vi "test_VIRefnumArray.vi"(8 "error in (no error)":errorcluster) -> (0 "error out":errorcluster)   [LabVIEW 2020]
uses:
  run-tests/Run Test (VIRefnum Array).vi
  Caraya.lvlib
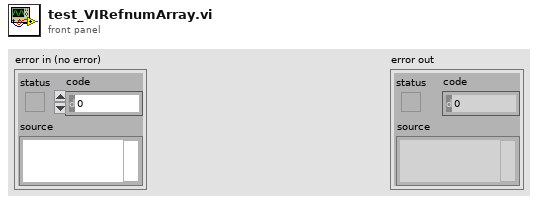
[diagram p1: front panel]
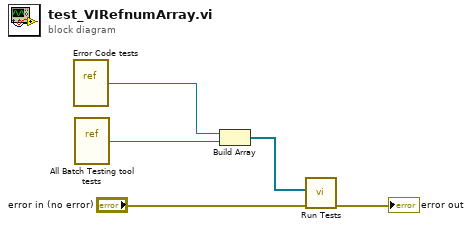
[diagram p0: block diagram]
diagram:
  n1 = vi-ref "Error Code tests.vi"() -> (w2:refnum<vi>)
  n2 = vi-ref "All Batch Testing tool tests.vi"() -> (w1:refnum<vi>)
  n3 = Build Array(w2, w1) -> (w3:refnum<vi>[])
  n4 = call-poly "Run Tests.vi"("error in"="error in (no error)", "VI Refnums"=w3) -> ("error out"=→"error out":errorcluster)  [unwired: 8 in, 1 out]
